vi "channel name sr name.vi"(8 "error constant":errorcluster, 11 "output Table":string[][](array[string])) -> (0 "error constant 2":errorcluster, 3 "Array":string[][](array[string]))   [LabVIEW 2018]
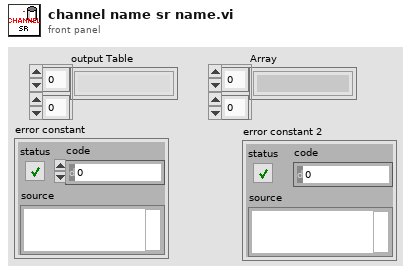
[diagram p1: front panel]
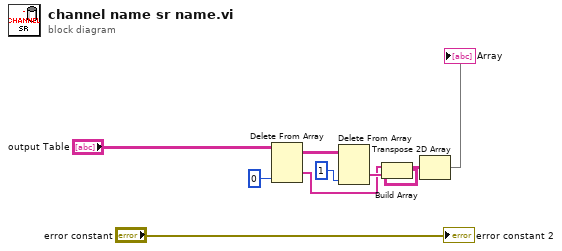
[diagram p0: block diagram]
diagram:
  n1 = Delete From Array(array="output Table", index (col)=0 ("disabled index (col)")) -> (deleted portion=w6:string[], array with subset deleted=w4:string[][])  [unwired: 2 in]
  n2 = Delete From Array(array=w4, index (col)=1 ("disabled index (col)")) -> (deleted portion=w7:string[])  [unwired: 2 in, 1 out]
  n3 = Build Array(w6, w7) -> (w8:string[][])
  n4 = Transpose 2D Array(2D array=w8) -> (transposed array=→"Array":string[][])
  "error constant 2" <- "error constant"
